vi "CPU_MEM_RAM.vi"(5 "read all":bool, 7 "oper":enum16{"init", "read", "write"}(ring), 10 "value in":u8 format="%02x", 11 "address":u16 format="%.0x") -> (2 "value out":u8 format="%02x", 3 "mem":u8[](array[numeric]))   [LabVIEW 2018]
panel:
  in  "init size":u16=65535 format="%.0x"
  # "used only for CPU test"
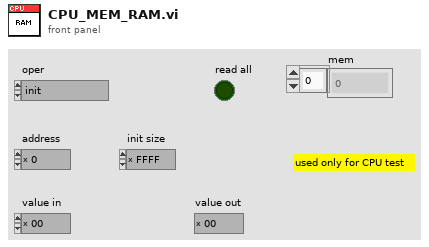
[diagram p1: front panel]
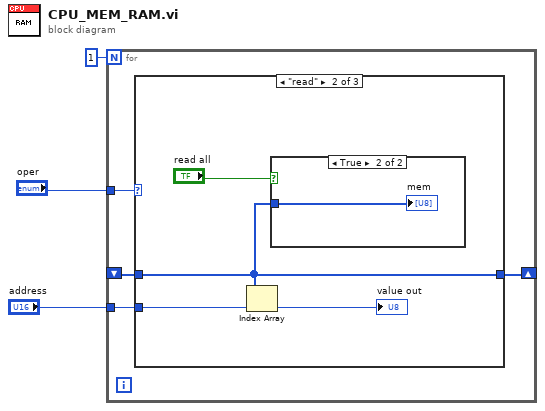
[diagram p0: block diagram]
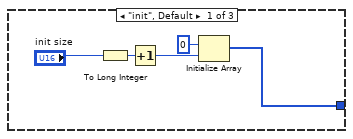
[diagram p2: hidden frame]
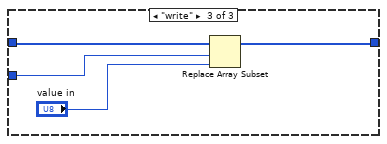
[diagram p4: hidden frame]
diagram:
  n1 = for {
    N: 1 -> [_]
    tunnel: "oper" -> [w7]
    tunnel: "address" -> [w6]
    shift-right: [w4] -> _
    shift-left: _ -> [w5]
    n2 = case shown="\"read\"" w7 {
      tunnel: w6 -> [_ w16 w19]
      tunnel: w5 -> [_ w15 w21]
      tunnel: [w9 w15 w20] -> w4
      frame "init", Default {
        n3 = To Long Integer(number="init size") -> (32bit integer=w10:i32)
        n4 = Increment(x=w10) -> (x+1=w11:i32)
        n5 = Initialize Array(u8 0 ("element"), w11) -> (w9:u8[])
      }
      frame "read" {
        n6 = Index Array(array=w15, index=w16) -> (element=→"value out":u8)
        n7 = case shown="True" "read all" {
          tunnel: w15 -> [_ w17]
          frame False {
          }
          frame True {
            "mem" <- w17
          }
        }
      }
      frame "write" {
        n8 = Replace Array Subset(array=w21, new element="value in", index=w19) -> (w20:u8[])
      }
    }
  }
